vi "niRFUtil RFHS CONV 1 Ohm Watt to dBm (real array).vi"(7 "Real Array (W)":T1 min=0 max=127 format="%.2f", 11 "error in (no error)":errorcluster) -> (8 "Real Array (dBm)":T1 min=0 max=127 format="%.2f", 13 "a":sgl, 14 "b":sgl=10.0, 15 "error out":errorcluster)   [LabVIEW 2015, in "niRFUtil.lvlib"]
doc: "(c) Copyright 2006, National Instruments, Inc. This VI may not be duplicated, sold, or distributed without written consent from National Instruments."
uses:
  niRFUtil.lvlib
  Includes/niRFUtil INC Real Array.ctl
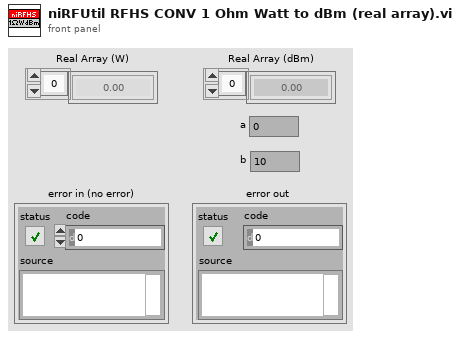
[diagram p1: front panel]
types:
  T1 = typedef "niRFUtil.lvlib/niRFUtil INC Real Array.ctl" = sgl[]
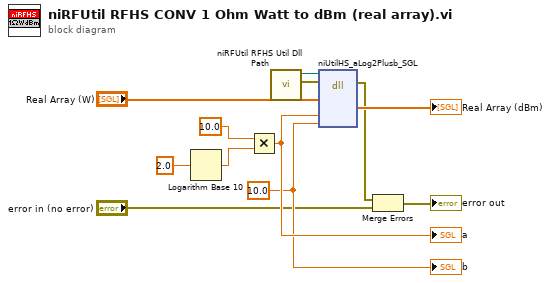
[diagram p0: block diagram]
diagram:
  w8 = sgl 10.0
  n1 = Logarithm Base 10(1:sgl 2.0 ("x")) -> (0:w10:sgl)
  n2 = Multiply(x=sgl 10.0, y=w10) -> (x*y=w9:sgl)
  "a" <- w9
  n3 = call "niRFUtil RFHS Util Dll Path.vi"() -> ("error out"=w6:errorcluster, "Path"=w7:path)  [unwired: 7 in, 3 out]
  n4 = dll-call lib="M:/RfProtocols/RFmx/DLLs/niRFHS/trunk/2.1/dist/win32U/niRFHS_avx.dll" fn="niUtilHS_aLog2Plusb_SGL" label="a*log2(x)+b"(path in=w7, error in=w6, "iBuf"="Real Array (W)", "a"=w9, "b"=w8) -> (error out=w2:errorcluster, "oBuf"=→"Real Array (dBm)":sgl[])  [unwired: 6 in, 1 out]
  n5 = Merge Errors(w2, "error in (no error)") -> (→"error out":errorcluster)
  "b" <- w8
